vi "Import Export - Initialize Dialog.vi"(8 "Error In":errorcluster, 10 "Tree Ctl Refnum":refnum<vi>, 11 "Item Ref in":T1 format="%.0x") -> (0 "Error Out":errorcluster, 1 "EC Master Found?":bool, 3 "Item Ref out":T1 format="%.0x")   [LabVIEW 2017, in "Scan Engine Custom Device.lvlib"]
uses:
  Scan Engine Custom Device.lvlib
  <vilib>/NI Veristand/Custom Device API/Custom Device Item Ref.ctl
  NationalInstruments.VeriStand.Internal
  Globals/Scan Engine GUIDs.vi
  <vilib>/NI Veristand/Custom Device API/Custom Device API.lvlib
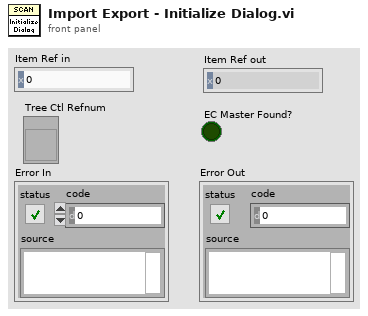
[diagram p1: front panel]
types:
  T1 = typedef "Custom Device API.lvlib/Custom Device Item Ref.ctl" = u64
  T2 = typedef "imagedata.ctl" = cluster{"image type":i32, "image depth":i32, "image":u8[], "mask":u8[], "colors":u32[], "Rectangle":cluster{"left":i16, "top":i16, "right":i16, "bottom":i16}}
  T3 = cluster{"Name":string, "GUID":string, "Tree Item Level":i32}[]
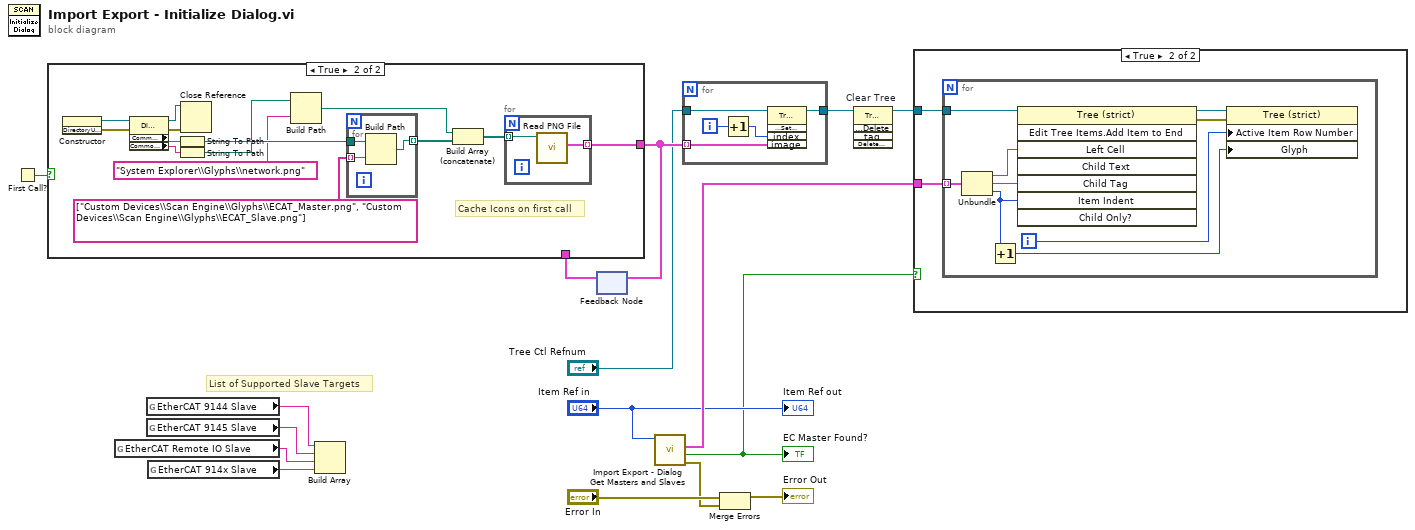
[diagram p0: block diagram]
diagram:
  # "List of Supported Slave Targets"
  n1 = First Call?() -> (First Call?: T/F=w7:bool)
  n2 = global read "Scan Engine GUIDs.vi" "EtherCAT Remote IO Slave"() -> (w12:string)
  n3 = global read "Scan Engine GUIDs.vi" "EtherCAT 9144 Slave"() -> (w14:string)
  n4 = global read "Scan Engine GUIDs.vi" "EtherCAT 9145 Slave"() -> (w13:string)
  n5 = global read "Scan Engine GUIDs.vi" "EtherCAT 914x Slave"() -> (w11:string)
  n6 = Build Array(w14, w13, w12, w11) -> ()  [unwired: 1 out]
  n7 = feedback #1() -> (w5:T2[])  [unwired: 1 in]
  n8 = case shown="True" w7 {
    tunnel: [w17 w18] -> w6
    tunnel: w5 -> [w17 _]
    frame False {
    }
    frame True {
      # "Cache Icons on first call"
      n9 = constructor class="DirectoryUtilities"() -> (reference out=w31:refnum<k24>, error out=w28:errorcluster)  [unwired: 3 in, 1 out]
      n10 = property class="DirectoryUtilities"(reference=w31, error in=w28) -> (reference out=w30:refnum<k24>, error out=w27:errorcluster, "CommmonDocuments"=w29:string, "CommonApplicationData"=w24:string)
      n11 = String To Path(string=w29) -> (path=w25:path)
      n12 = String To Path(string=w24) -> (path=w23:path)
      n13 = Close Reference(reference=w30, error in (no error)=w27) -> ()  [unwired: 1 out]
      n14 = Build Path(base path=w23, name or relative path="System Explorer\\Glyphs\\network.png") -> (appended path=w20:path)
      n15 = for {
        tunnel: string[] ["Custom Devices\\Scan Engine\\Glyphs\\ECAT_Master.png", "Custom Devices\\Scan Engine\\Glyphs\\ECAT_Slave.png"] -> [w36] mode=indexing
        tunnel: w25 -> [w35]
        tunnel: [w34] -> w21 mode=indexing
        n16 = Build Path(base path=w35, name or relative path=w36) -> (appended path=w34:path)
      }
      n17 = Build Array (concatenate)(w20, w21) -> (w19:path[])
      n18 = for {
        tunnel: w19 -> [w33] mode=indexing
        tunnel: [w32] -> w18 mode=indexing
        n19 = call <vilib>:"Read PNG File.vi"("path to PNG file"=w33) -> ("image data"=w32:T2)  [unwired: 8 in, 2 out]
      }
    }
  }
  n20 = feedback-in #1(w6) -> ()
  n21 = call "Import Export - Dialog Get Masters and Slaves.vi"("Item Ref in"="Item Ref in") -> ("error out"=w8:errorcluster, "EC Master Found?"=w1:bool, "EC Master And Slaves"=w3:T3)  [unwired: 7 in, 1 out]
  "EC Master Found?" <- w1
  n22 = for {
    tunnel: "Tree Ctl Refnum" -> [w41]
    tunnel: [w40] -> w9
    tunnel: w6 -> [w37] mode=indexing
    i -> [w39]
    n23 = Increment(x=w39) -> (x+1=w38:i32)
    n24 = invoke on="Invoke Node" class="Tree (strict)" method="Custom Item Symbols.Set Symbol"(reference=w41, "index"=w38, "image"=w37) -> (reference out=w40:refnum<vi>)  [unwired: 2 in, 4 out]
  }
  n25 = Merge Errors("Error In", w8) -> (→"Error Out":errorcluster)
  n26 = invoke on="Clear Tree" class="Tree (strict)" method="Edit Tree Items.Delete"(reference=w9) -> (reference out=w10:refnum<vi>)  [unwired: 4 in, 4 out]
  n27 = case shown="True" w1 {
    tunnel: w10 -> [_ w43]
    tunnel: w3 -> [_ w42]
    frame False {
    }
    frame True {
      n28 = for {
        tunnel: w43 -> [w52]
        tunnel: w42 -> [w51] mode=indexing
        i -> [w45]
        n29 = Unbundle(w51) -> ("Name"=w50:string, "GUID"=w49:string, "Tree Item Level"=w46:i32)
        n30 = Increment(x=w46) -> (x+1=w44:i32)
        n31 = invoke on="Invoke Node" class="Tree (strict)" method="Edit Tree Items.Add Item to End"(reference=w52, "Left Cell"=w50, "Child Tag"=w49, "Item Indent"=w46) -> (reference out=w48:refnum<vi>, error out=w47:errorcluster)  [unwired: 4 in, 6 out]
        n32 = property class="Tree (strict)"(reference=w48, error in=w47, "Active Item Row Number"=w45, "Glyph"=w44) -> ()  [unwired: 2 out]
      }
    }
  }
  "Item Ref out" <- "Item Ref in"
